vi "septimo.vi"() -> ()   [LabVIEW 2012]
panel:
  out "Numeric":i32
  in  "stop":bool
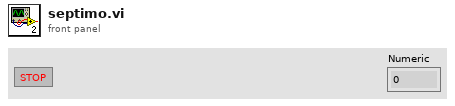
[diagram p1: front panel]
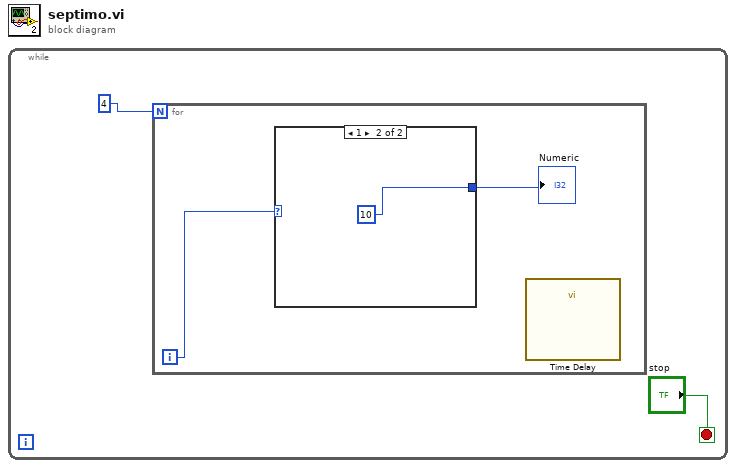
[diagram p0: block diagram]
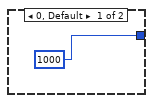
[diagram p2: hidden frame]
diagram:
  n1 = while {
    stop <- "stop" stop-if-true
    n2 = for {
      N: 4 -> [_]
      i -> [w4]
      n3 = case shown="1" w4 {
        tunnel: [1000 10] -> w3
        frame 0, Default {
        }
        frame 1 {
        }
      }
      "Numeric" <- w3
      n4 = call "Time Delay"() -> ()  [unwired: 11 in, 1 out]
    }
  }
